vi "Query Faults.vi"(7 "Slave Address":i32=-1 min=-1 max=30 step=1, 8 "error":errorcluster, 11 "VISA":refnum<visa-resource-name>) -> (0 "error out":errorcluster, 1 "Number":u32, 2 "Fault?":bool, 3 "VISA out":refnum<visa-resource-name>, 4 "Descriptions":string[](array[string]))   [LabVIEW 2019, in "TDK-Lambda GEN LAN Series.lvlib"]
doc: "Reads the power supply's questionable condition register (\"STAT:QUES:COND?\") to find any instrument faults. A fault condition will shut the instrument output off and display an error message on it's front panel. \n\nThe returned indicators include:\n- Fault: TRUE if fault condition exists and output is off.\n- Number: integer value of Questionable Condition register.\n- Descriptions: array of strings. Shows description of all active faults. \n Size of the array equals the number of faults. \n\nSee the Genesys LAN User Manual for a description of faults."
uses:
  <instrlib>/TDK-Lambda GEN LAN Series/TDK-Lambda GEN LAN Series.lvlib
panel:
  # "TDK-Lambda Genesys \n LAN\n  DC Power Supplies"
  # "Read if Fault Occurred"
  # "(c) 2019 TDK-Lambda.  ALL RIGHTS RESERVED."
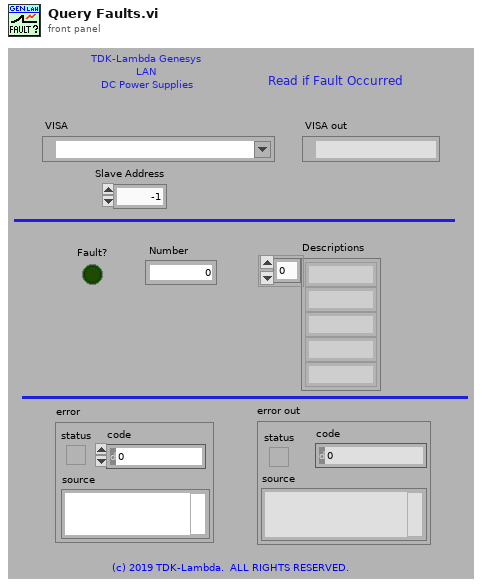
[diagram p1: front panel]
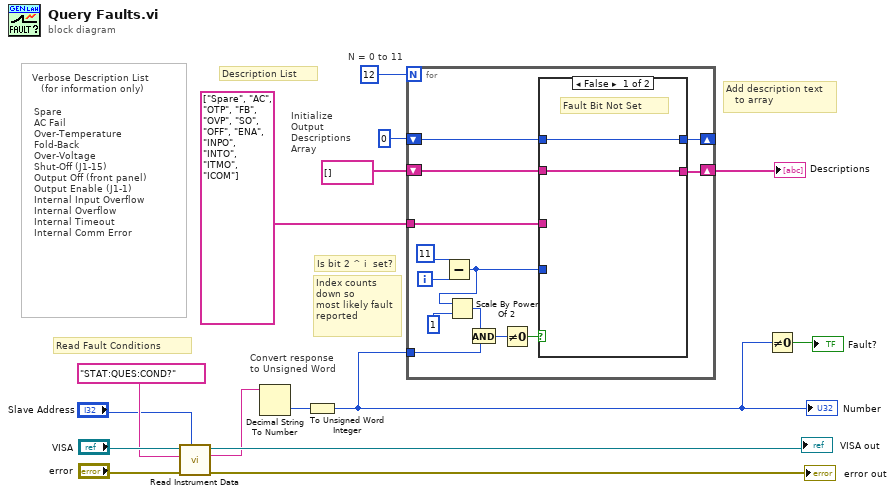
[diagram p0: block diagram]
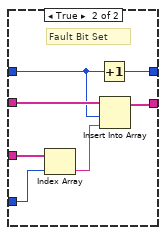
[diagram p2: hidden frame]
diagram:
  # "Spare\nAC Fail\nOver-Temperature\nFold-Back\nOver-Voltage\nShut-Off (J1-15)\nOutput Off (front panel)\nOutput Enable (J1-1)\nInternal Input Overflow\nInternal Overflow\nInternal Timeout\nInternal Comm Error"
  # "Verbose Description List \n   (for information only)"
  # "Initialize\nOutput\nDescriptions\nArray"
  # "Add description text \n   to array"
  # "Index counts\ndown so\nmost likely fault\nreported"
  # "Is bit 2 ^ i  set?"
  # "N = 0 to 11"
  # "Convert response\nto Unsigned Word"
  # "Description List"
  # "Read Fault Conditions"
  n1 = call <instrlib>:"Read Instrument Data.vi"("Slave Address"="Slave Address", "error"="error", "Query"="STAT:QUES:COND?" ("format string"), "VISA"="VISA") -> ("error out"=→"error out":errorcluster, "Response"=w13:string, "VISA out"=→"VISA out":refnum<visa-resource-name>)  [unwired: 4 in, 1 out]
  n2 = Decimal String To Number(string=w13) -> (number=w12:i32)  [unwired: 2 in, 1 out]
  n3 = To Unsigned Word Integer(number=w12) -> (unsigned 16bit integer=w2:u16)
  "Number" <- w2
  n4 = for {
    N: 12 -> [_]
    tunnel: w2 -> [w26]
    tunnel: string[] ["Spare", "AC", "OTP", "FB", "OVP", "SO", "OFF", "ENA", "INPO", "INTO", "ITMO", "ICOM"] ("Descriptions") -> [w20]
    shift-right: [w16] -> w5
    shift-left: string[] [] ("Descriptions") -> [w17]
    shift-right: [w18] -> _
    shift-left: 0 -> [w19]
    i -> [w22]
    n5 = Subtract(x=11, y=w22) -> (x-y=w21:i32)
    n6 = Scale By Power Of 2(n=w21, x=u16 1) -> (x*2^n=w24:u16)
    n7 = And(x=w24, y=w26) -> (x .and. y?=w27:u16)
    n8 = Not Equal To 0?(x=w27) -> (x != 0?=w25:bool)
    n9 = case shown="False" w25 {
      tunnel: w21 -> [_ w37]
      tunnel: w20 -> [_ w36]
      tunnel: w19 -> [w30 w31]
      tunnel: [w30 w34] -> w18
      tunnel: w17 -> [w29 w33]
      tunnel: [w29 w32] -> w16
      frame False {
        # "Fault Bit Not Set"
      }
      frame True {
        # "Fault Bit Set"
        n10 = Index Array(array=w36, index=w37) -> (element=w35:string)
        n11 = Increment(x=w31) -> (x+1=w34:i32)
        n12 = Insert Into Array(array=w33, index=w31, new element=w35) -> (w32:string[])
      }
    }
  }
  "Descriptions" <- w5
  n13 = Not Equal To 0?(x=w2) -> (x != 0?=→"Fault?":bool)
